vi "Generator&oscilloscope.vi"() -> ()   [LabVIEW 2018]
uses:
  <instrlib>/LeCroy Wave Series/Public/Data/Read Single Waveform.vi
  <instrlib>/Siglent SDG X Series/Siglent SDG X Series.lvlib
  <instrlib>/LeCroy Wave Series/LeCroy Wave Series.lvlib
panel:
  in  "Stop":bool
  in  "Tab Control":enum32{"Page 1", "Page 2"}(tab)
  in  "VISA Refnum in":refnum<visa-resource-name>
  in  "error in (no error)":errorcluster
  in  "Channel (1:Channel 1)":i32(ring)=1 items=["Channel 1"=1, "Channel 2"=2]
  in  "Enable Output (T: Enable)":bool=TRUE
  in  "Amplitude (1.0 Vpp)":dbl=1.0 format="%#.3f"
  in  "Frequency (1000 Hz)":dbl=1000.0 format="%#.6g"
  in  "DC Offset (0.00 V) in":dbl
  in  "Waveform Function (0: Sine) in":u16(ring) items=["Sine", "Square", "Ramp", "DC", "Pulse", "Arb"]
  in  "Phase (0.0 degrees)":dbl=0.002 min=-360.0 max=360.0 format="%#.1g"
  in  "Fall (20 ns)":dbl=2e-08 format="%#.3g"
  in  "Duty (20%)":dbl=20.0 min=0.0001 max=100.0 format="%.4g"
  in  "Delay (0.00 s)":dbl min=-1000000.0 max=1000000.0
  in  "Rise (20 ns)":dbl=2e-08 format="%#.3g"
  in  "True To \ngenerate\n pulse":bool
  out "VISA resource name out":refnum<visa-resource-name>
  out "error out":errorcluster
  in  "format string":string
  out "Output Filename":path
  out "error out 2":errorcluster
  in  "Filename":string="filename"
  in  "Path":string="c:\\path structure\\"
  out ".not. x?":bool
  in  "stop":bool
  out "Waveform Data":waveform(dbl)(graph)
  in  "Timeout (10000 ms)":u32=10000
  in  "Source (0: Channel 1)":u16(ring) items=["Channel 1", "Channel 2", "Channel 3", "Channel 4", "Memory 1", "Memory 2", "Memory 3", "Memory 4", "Function 1", "Function 2", "Function 3", "Function 4", "Function 5", "Function 6", "Function 7", "Function 8"]
  in  "Perform Auto Setup?":bool
  in  "Reset Scope?":bool
  in  "VISA resource name":refnum<visa-resource-name>
  out "Saved filename":string
  # "Set PULSE parameters"
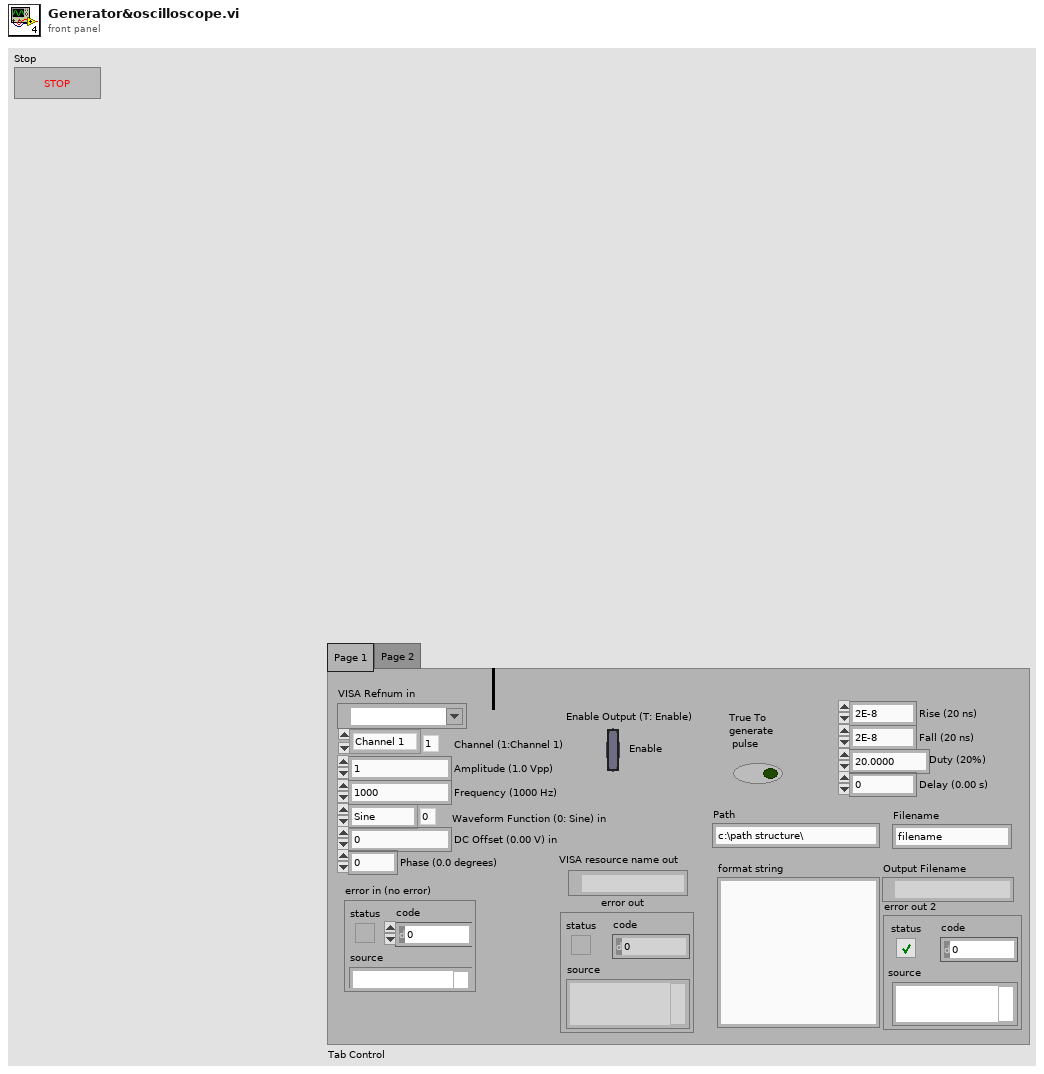
[diagram p1: front panel]
types:
  T1 = enum16{"open", "replace", "create", "open or create", "replace or create", "replace or create with confirmation"}
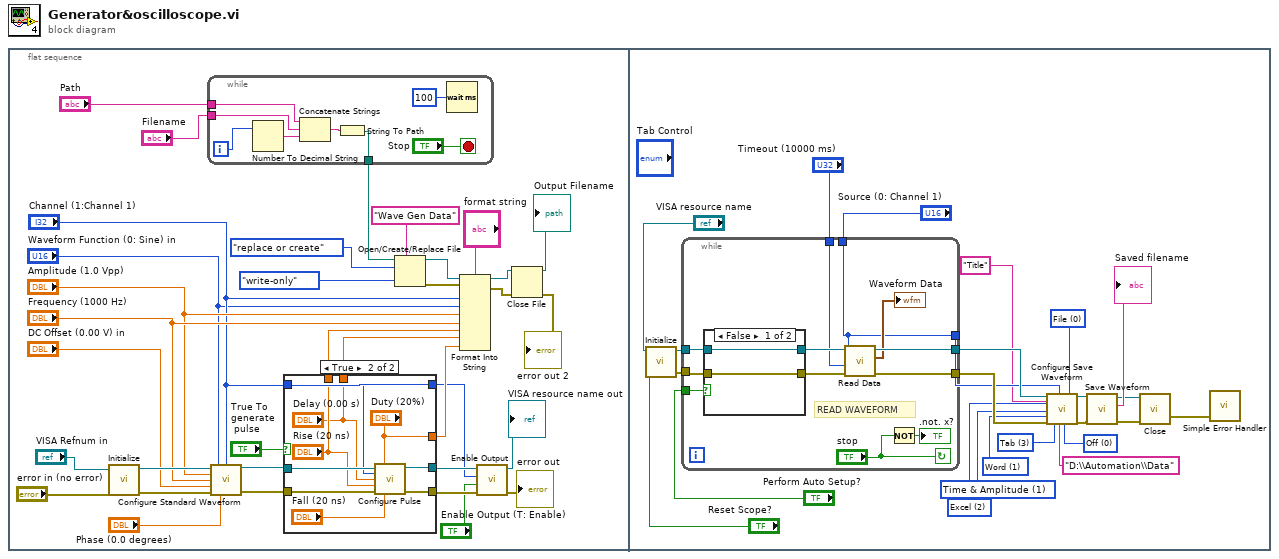
[diagram p0: block diagram]
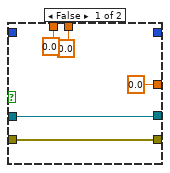
[diagram p2: hidden frame]
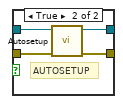
[diagram p3: hidden frame]
diagram:
  n1 = flat-sequence {
    frame #0 {
      n2 = call <instrlib>:"Initialize.vi"("error in (no error)"="error in (no error)", "VISA resource name"="VISA Refnum in") -> ("error out"=w28:errorcluster, "VISA resource name out"=w29:refnum<visa-resource-name>)  [unwired: 8 in]
      n3 = while {
        tunnel: "Path" -> [w37]
        tunnel: "Filename" -> [w36]
        tunnel: [w35] -> w1
        i -> [w41]
        stop <- "Stop" stop-if-true
        n4 = Number To Decimal String(number=w41) -> (decimal integer string=w42:string)  [unwired: 1 out]
        n5 = Concatenate Strings(w37, w36, w42) -> (w40:string)
        n6 = String To Path(string=w40) -> (path=w35:path)
        n7 = Wait (ms)(milliseconds to wait=u32 100) -> ()  [unwired: 1 out]
      }
      n8 = call <instrlib>:"Configure Standard Waveform.vi"("VISA resource name"=w29, "Waveform Function (0: Sine)"="Waveform Function (0: Sine) in", "Channel (1:Channel 1)"="Channel (1:Channel 1)", "Amplitude (1.0 Vpp)"="Amplitude (1.0 Vpp)", "Frequency (1000 Hz)"="Frequency (1000 Hz)", "DC Offset (0.00 V)"="DC Offset (0.00 V) in", "error in (no error)"=w28, "Phase (0.0 degrees)"="Phase (0.0 degrees)") -> ("VISA resource name out"=w24:refnum<visa-resource-name>, "error out"=w27:errorcluster)  [unwired: 6 in]
      n9 = case shown="True" "True To \ngenerate\n pulse" {
        tunnel: [w47 w55] -> w34
        tunnel: [w46 w54] -> w33
        tunnel: w24 -> [w47 w53]
        tunnel: w27 -> [w46 w52]
        tunnel: "Channel (1:Channel 1)" -> [_ w51]
        tunnel: "Channel (1:Channel 1)" -> [_ _]
        tunnel: [0.0 ("Duty (20%)") "Duty (20%)"] -> w16
        tunnel: [0.0 ("Rise (20 ns)") "Rise (20 ns)"] -> w7
        tunnel: [0.0 ("Delay (0.00 s)") "Delay (0.00 s)"] -> w6
        frame False {
        }
        frame True {
          n10 = call <instrlib>:"Configure Pulse.vi"("VISA resource name"=w53, "Duty (20%)"="Duty (20%)", "Channel (1:Channel 1)"=w51, "Delay (0.00 s)"="Delay (0.00 s)", "Rise (20 ns)"="Rise (20 ns)", "error in (no error)"=w52, "Fall (20 ns)"="Fall (20 ns)") -> ("VISA resource name out"=w55:refnum<visa-resource-name>, "error out"=w54:errorcluster)  [unwired: 7 in]
        }
      }
      n11 = Open/Create/Replace File(file path (use dialog)=w1, prompt="Wave Gen Data", operation (0:open)=T1."replace or create", access (0:read/write)=enum16{"read/write", "read-only", "write-only"}."write-only") -> (refnum out=w18:refnum<file>, error out=w19:errorcluster)  [unwired: 2 in, 1 out]
      n12 = Format Into String(format string="format string", initial string=w18, error in=w19, "Channel (1:Channel 1)", "Waveform Function (0: Sine) in", "Amplitude (1.0 Vpp)", "Frequency (1000 Hz)", w7, w6, w16) -> (resulting string=w14:refnum<file>, error out=w11:errorcluster)
      n13 = call <instrlib>:"Enable Output.vi"("error in (no error)"=w33, "Enable Output (T: Enable)"="Enable Output (T: Enable)", "Channel (1:Channel 1)"="Channel (1:Channel 1)", "VISA resource name"=w34) -> ("error out"=→"error out":errorcluster, "VISA resource name out"=→"VISA resource name out":refnum<visa-resource-name>)  [unwired: 6 in]
      n14 = Close File(refnum=w14, error in=w11) -> (path=→"Output Filename":path, error out=→"error out 2":errorcluster)
    }
    frame #1 {
      w63 = u16 3 items=["Comma", "Space", "Semicolon", "Tab"] ("Delimiter (  0:Comma)")
      w64 = u16 0 items=["Off", "Wrap", "Fill"] ("Auto Save (0:Off")
      w65 = u16 1 items=["Byte", "Word", "Auto"] ("BinarySubFormat (1: Word)")
      w67 = u16 1 items=["Amplitude Only", "Time & Amplitude", "With Header"] ("SubFormat (1: Time & Amplitude)")
      w68 = u16 2 items=["Binary", "ASCII", "Excel", "MATLAB", "MathCad", "WaveML"] ("Format (0: Binary)")
      w69 = u16 0 items=["File", "M1", "M2", "M3", "M4"] ("Destination (0:File)")
      n15 = call <instrlib>:"Initialize.vi"("Reset? (T: Yes)"="Reset Scope?", "VISA resource name"="VISA resource name") -> ("error out"=w77:errorcluster, "VISA resource name out"=w78:refnum<visa-resource-name>)  [unwired: 8 in]
      n16 = while {
        tunnel: [w90] -> w71
        tunnel: [w89] -> w72
        tunnel: "Perform Auto Setup?" -> [w88]
        tunnel: "Source (0: Channel 1)" -> [w81]
        tunnel: w77 -> [w87]
        tunnel: w78 -> [w86]
        tunnel: "Timeout (10000 ms)" -> [w85]
        tunnel: [w81] -> w70
        stop <- "stop" continue-if-true
        # "READ WAVEFORM"
        n17 = case shown="False" w88 {
          tunnel: w87 -> [w93 w98]
          tunnel: w86 -> [w94 w97]
          tunnel: [w94 w96] -> w92
          tunnel: [w93 w95] -> w91
          frame False {
          }
          frame True {
            # "AUTOSETUP"
            n18 = call <instrlib>:"Autosetup.vi"("error in (no error)"=w98, "VISA resource name"=w97) -> ("error out"=w95:errorcluster, "VISA resource name out"=w96:refnum<visa-resource-name>)  [unwired: 8 in]
          }
        }
        n19 = call-poly <instrlib>:"Read Data.vi"("error in (no error)"=w91, "Timeout (10000 ms)"=w85, "Source (0: Channel 1)"=w81, "VISA resource name"=w92) -> ("error out"=w90:errorcluster, "Waveform Data"=→"Waveform Data":waveform(dbl), "VISA resource name out"=w89:refnum<visa-resource-name>)  [unwired: 5 in]
        n20 = Not(x="stop") -> (.not. x?=→".not. x?":bool)
      }
      n21 = call <instrlib>:"Configure Save Waveform.vi"("VISA resource name"=w72, "Trace Title (Title)"="Title", "Format (0: Binary)"=w68, "SubFormat (1: Time & Amplitude)"=w67, "BinarySubFormat (1: Word)"=w65, "error in (no error)"=w71, "Delimiter (  0:Comma)"=w63, "Source (0: Channel 1)"=w70, "Save Files in Directory (D:\\Waveforms)"="D:\\Automation\\Data" ("Save Files in Directory (D:\\Waveforms)"), "Auto Save (0:Off"=w64, "Destination (0:File)"=w69) -> ("VISA resource name out"=w61:refnum<visa-resource-name>, "error out"=w60:errorcluster)  [unwired: 7 in]
      n22 = call <instrlib>:"Save Waveform.vi"("error in (no error)"=w60, "VISA resource name"=w61) -> ("error out"=w57:errorcluster, "Saved filename"=→"Saved filename":string, "VISA resource name out"=w58:refnum<visa-resource-name>)  [unwired: 7 in]
      n23 = call <instrlib>:"Close.vi"("error in (no error)"=w57, "VISA resource name"=w58) -> ("error out"=w80:errorcluster)  [unwired: 9 in]
      n24 = call <vilib>:"Simple Error Handler.vi"("error in (no error)"=w80) -> ()  [unwired: 4 in, 5 out]
    }
  }
